vi "Record Data Return Failure.vi"(5 "Base Reported Value":dbl, 7 "Reported Value":string, 8 "error in (no error)":errorcluster, 9 "Column":i32, 10 "Row":i32, 11 "report in":refnum<class "NI_report.lvclass">) -> (0 "error out":errorcluster, 1 "Repeat?":bool, 2 "Row Out":i32, 3 "report out":refnum<class "NI_report.lvclass">)   [LabVIEW 2019]
doc: "Used for recording As Found or As Left data to a Tektronix Data Report.\nReport In: Data Report to write data to\nRow: Excel Row (Zero Index)\nColumn: Excel Column (Zero Index)\nBase Reported Value: Numerical value obtained from measurement device. \n Devices report in Base Units. This value will be corrected to \n match the units on the data report for the Row given.\nReported Value: String to be written as is to the Data Report\nRow Out: The next row to be written to.\nRepeat?: If the recorded data is reported as a failure, and the user \n chooses to repeat the test, this will be TRUE, otherwise this \n will be FLASE."
uses:
  <vilib>/Utility/NIReport.llb/NI_report.lvclass
  <vilib>/addons/_office/_exclsub.llb/font.ctl
  <vilib>/addons/_office/excel.llb/Excel Get Data (str).vi
  <vilib>/addons/_office/NI_ReportGenerationToolkit.lvlib
  <vilib>/Utility/NIReport.llb/Excel/NI_Excel.lvclass
panel:
  out "column":i32
  out "Pass/Fail":string
  out "Balance Failure":bool=TRUE
  out "row":i32
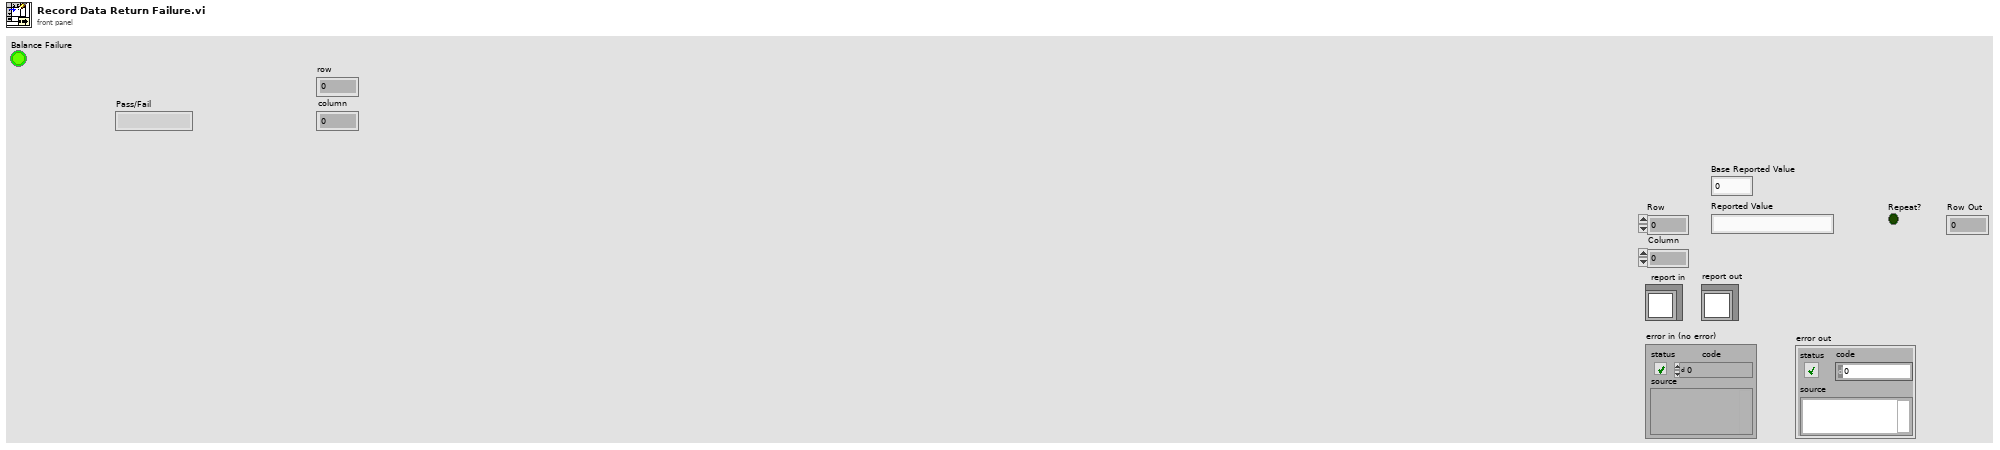
[diagram p1: front panel]
types:
  T1 = typedef "NI_ReportGenerationToolkit.lvlib/font.ctl" = cluster{"font name":string, "font size":dbl, "bold":u16, "italic":u16, "underline":u16, "strike through":u16, "font color":u32}
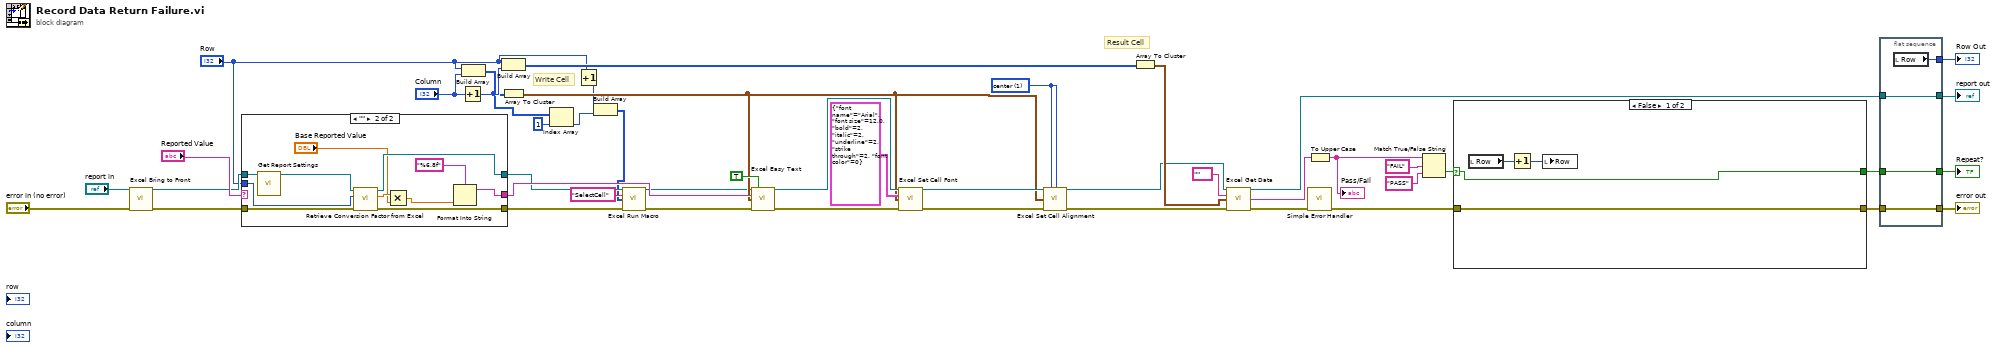
[diagram p0: block diagram]
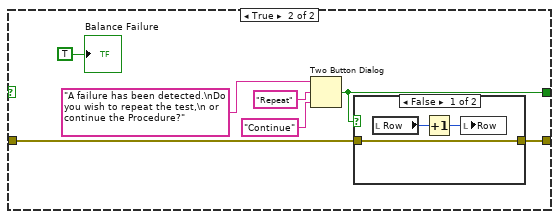
[diagram p3: hidden frame]
diagram:
  w21 = 1 items=["left", "center", "right"] ("horizontal alignment (left)")
  # "Result Cell"
  # "Write Cell"
  n1 = call <vilib>:"Excel Bring to Front.vi"("report in"="report in", "error in (no error)"="error in (no error)") -> ("report out"=w13:refnum<class "NI_report.lvclass">, "error out"=w17:errorcluster)  [unwired: 12 in]
  n2 = case shown="\"\"" "Reported Value" {
    selector: "Reported Value" -> [w49 _]
    tunnel: [w49 w53] -> w30
    tunnel: w17 -> [w48 w58]
    tunnel: "Row" -> [_ w57]
    tunnel: w13 -> [w47 w51]
    tunnel: [w47 w55] -> w12
    tunnel: [w48 w54] -> w10
    frame "False", Default {
    }
    frame "" {
      n3 = call-dynamic "Get Report Settings.vi"("report in"=w51) -> ("report out"=w50:refnum<class "NI_report.lvclass">)  [unwired: 10 in, 4 out]
      n4 = call <userlib>:"Retrieve Conversion Factor from Excel.vi"("error in (no error)"=w58, "Row"=w57, "report in"=w50) -> ("error out"=w54:errorcluster, "Conversion factor"=w56:dbl, "report out"=w55:refnum<class "NI_report.lvclass">)  [unwired: 6 in]
      n5 = Multiply(x=w56, y="Base Reported Value") -> (x*y=w59:dbl)
      n6 = Format Into String(format string="%6.8f", w59) -> (resulting string=w53:string)  [unwired: 2 in, 1 out]
    }
  }
  n7 = Increment(x="Column") -> (x+1=w46:i32)
  n8 = Build Array("Row", "Column") -> (w6:i32[])
  n9 = Build Array("Row", w46) -> (w7:i32[])
  n10 = Array To Cluster(array=w6) -> (cluster=w18:cluster{"[0]":i32, "[1]":i32})
  n11 = Index Array(array=w6, index=1) -> (element=w4:i32)
  n12 = Increment(x="Row") -> (x+1=w2:i32)
  n13 = Build Array(w2, w4) -> (w1:i32[])
  n14 = call <vilib>:"Excel Run Macro.vi"("report in"=w12, "macro name"="SelectCell", "parameters"=w1, "error in (no error)"=w10) -> ("report out"=w11:refnum<class "NI_report.lvclass">, "error out"=w9:errorcluster)  [unwired: 9 in, 1 out]
  n15 = call <vilib>:"Excel Easy Text.vi"("report in"=w11, "border? (F)"=TRUE, "text"=w30, "start (-1, -1)"=w18, "error in (no error)"=w9) -> ("report out"=w26:refnum<class "NI_report.lvclass">, "error out"=w25:errorcluster)  [unwired: 6 in, 3 out]
  n16 = call <vilib>:"Excel Set Cell Font.vi"("report in"=w26, "font"=T1 {"font name"="Arial", "font size"=12.0, "bold"=2, "italic"=2, "underline"=2, "strike through"=2, "font color"=0}, "start (-1, -1)"=w18, "error in (no error)"=w25) -> ("report out"=w24:refnum<class "NI_report.lvclass">, "error out"=w23:errorcluster)  [unwired: 10 in]
  n17 = call <vilib>:"Excel Set Cell Alignment.vi"("report in"=w24, "vertical alignment (top)"=w21, "horizontal alignment (left)"=w21, "start (-1, -1)"=w18, "error in (no error)"=w23) -> ("report out"=w20:refnum<class "NI_report.lvclass">, "error out"=w19:errorcluster)  [unwired: 9 in]
  n18 = Array To Cluster(array=w7) -> (cluster=w22:cluster{"[0]":i32, "[1]":i32})
  n19 = call-poly <vilib>:"Excel Get Data.vi"("report in"=w20, "data type"="", "start (0, 0)"=w22, "error in (no error)"=w19) -> ("report out"=w38:refnum<class "NI_report.lvclass">, "data"=w45:string, "error out"=w29:errorcluster)  [unwired: 9 in]
  n20 = To Upper Case(1:w45) -> (0:w44:string)
  "Pass/Fail" <- w44
  n21 = call <vilib>:"Simple Error Handler.vi"("error in (no error)"=w29) -> ("error out"=w41:errorcluster)  [unwired: 4 in, 4 out]
  n22 = Match True/False String(2:"PASS" ("false string"), 3:"FAIL" ("true string"), 4:w44) -> (0:w42:bool)  [unwired: 1 out]
  n23 = case shown="False" w42 {
    selector: w42 -> [w64 _]
    tunnel: [w64 w68] -> w36
    tunnel: [w63 w67] -> w34
    tunnel: w41 -> [w63 w66]
    frame False {
      n24 = local read "Row"() -> (w61:i32)
      n25 = Increment(x=w61) -> (x+1=w62:i32)
      n26 = local write "Row"(w62) -> ()
    }
    frame True {
      n27 = Two Button Dialog(message="A failure has been detected.\nDo you wish to repeat the test,\n or continue the Procedure?", 1:"Continue" ("F button name (\"Cancel\")"), 2:"Repeat" ("T button name (\"OK\")")) -> (T button?=w68:bool)
      n28 = case shown="False" w68 {
        tunnel: [w74 w75] -> w67
        tunnel: w66 -> [w74 w75]
        frame False {
          n29 = local read "Row"() -> (w72:i32)
          n30 = Increment(x=w72) -> (x+1=w73:i32)
          n31 = local write "Row"(w73) -> ()
        }
        frame True {
        }
      }
      "Balance Failure" <- TRUE
    }
  }
  n32 = flat-sequence {
    tunnel: [w79] -> w37
    tunnel: w38 -> [w79]
    tunnel: [w78] -> w35
    tunnel: w36 -> [w78]
    tunnel: [w77] -> w33
    tunnel: w34 -> [w77]
    tunnel: [w76] -> w32
    frame #0 {
      n33 = local read "Row"() -> (w76:i32)
    }
  }
  "report out" <- w37
  "error out" <- w33
  "Repeat?" <- w35
  "Row Out" <- w32
